vi "VarD.vi"(2 "RCW (X2)":dbl(slide) scale=-1.0..1.0, 3 "FWD (Y)":dbl(slide) scale=-1.0..1.0, 4 "R":dbl, 5 "W":dbl) -> (0 "x = 0?":bool, 1 "D":dbl)   [LabVIEW 2013]
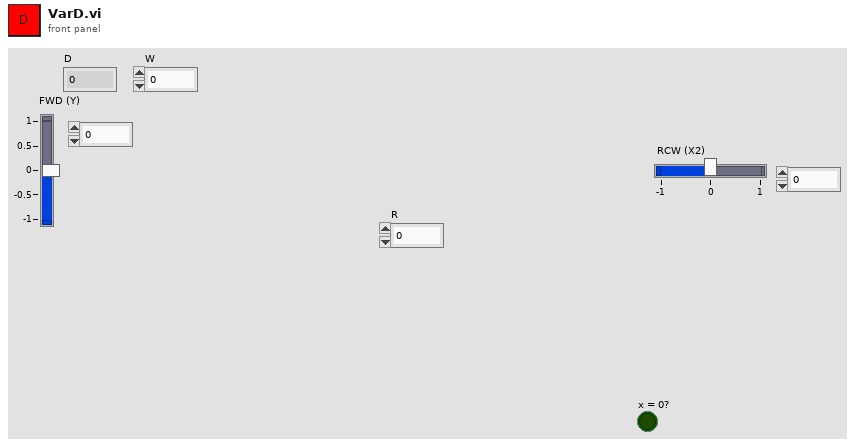
[diagram p1: front panel]
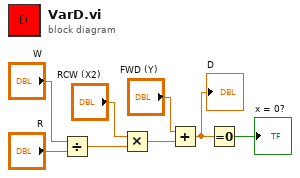
[diagram p0: block diagram]
diagram:
  n1 = Divide(x="W", y="R") -> (x/y=w7:dbl)
  n2 = Multiply(x="RCW (X2)", y=w7) -> (x*y=w3:dbl)
  n3 = Add(x="FWD (Y)", y=w3) -> (x+y=w1:dbl)
  "D" <- w1
  n4 = Equal To 0?(x=w1) -> (x = 0?=→"x = 0?":bool)
